vi "OP400ZP_SCANequipements.vi"(8 "Errin":errorcluster caption="errin", 10 "Chaîne":string="Log et conf\\Config.ini", 11 "pathin":path=path "D:/CODE/02 SLIM ZEN") -> (0 "errout":errorcluster={"status"=TRUE, "code"=0, "source"="PCAN_CHANNEL ILLEGAL"}, 1 "KO?":bool=TRUE, 4 "BT":refnum<visa-resource-name>, 6 "MX":refnum<visa-resource-name>)   [LabVIEW 2020]
doc: "Ce vi il détecte la presence des équipements"
uses:
  VG/VG_MX5060.vi
  VG/VG_BT3562.vi
  VG/VG_ARDUINO.vi
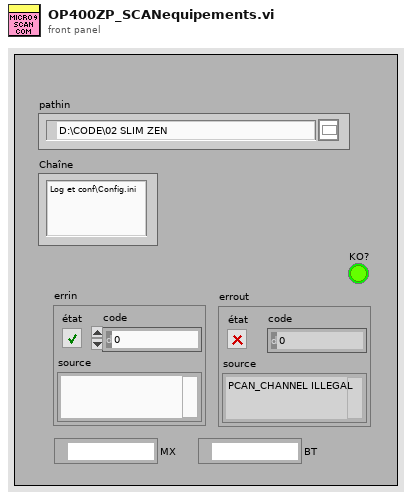
[diagram p1: front panel]
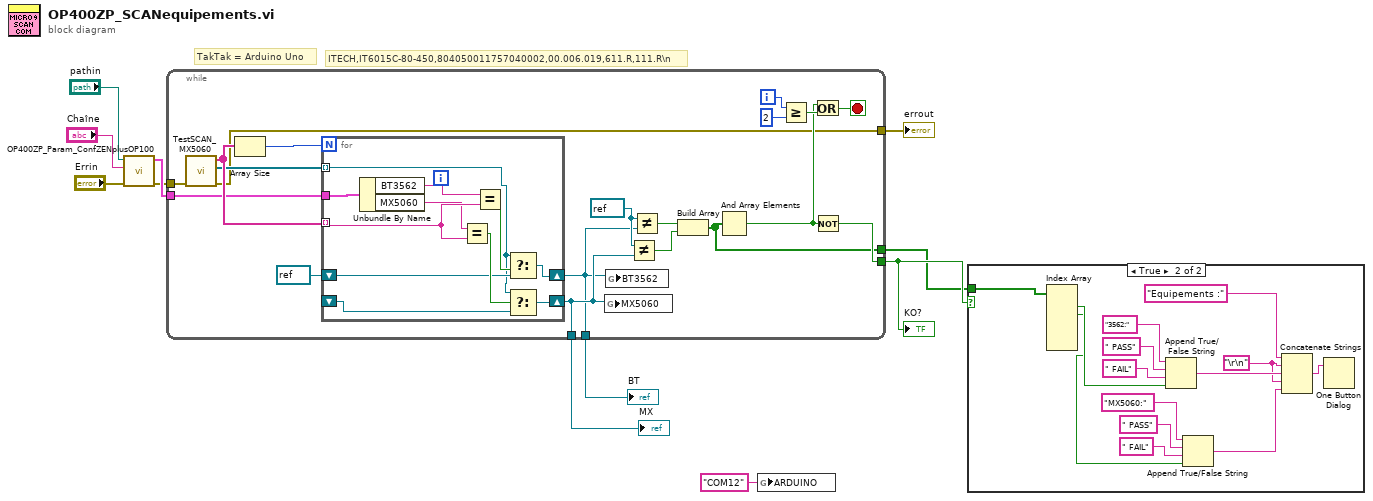
[diagram p0: block diagram]
diagram:
  # "TakTak = Arduino Uno"
  # "ITECH,IT6015C-80-450,804050011757040002,00.006.019,611.R,111.R\\n"
  n1 = call "OP400ZP_Param_ConfZENplusOP100.vi"("errin"="Errin", "Chaîne"="Chaîne", "pathin"="pathin") -> ("errout"=w8:errorcluster, "VISA OUT"=w9:cluster{"BT3562":string, "MX5060":string})  [unwired: 7 in]
  n2 = while {
    tunnel: w8 -> [w29]
    tunnel: [w24] -> w11
    tunnel: w9 -> [w21]
    tunnel: [w12] -> w10
    tunnel: [w18] -> w2
    tunnel: [w16] -> w4
    tunnel: [w15] -> w3
    i -> [w23]
    stop <- w26 stop-if-true
    w17 = refnum<visa-resource-name> refnum ("x")
    n3 = call "TestSCAN_MX5060.vi"("errin"=w29) -> ("error out"=w18:errorcluster, "Tableau 2"=w27:refnum<visa-resource-name>[], "Tableau"=w28:string[])  [unwired: 8 in]
    n4 = Array Size(array=w28) -> (size(s)=w30:i32)
    n5 = for {
      N: w30 -> [_]
      shift-right: [w40] -> w15
      shift-left: refnum<visa-resource-name> refnum ("VISA resource name out") -> [w34]
      tunnel: w28 -> [w37] mode=indexing
      tunnel: w27 -> [w31] mode=indexing
      tunnel: w21 -> [w39]
      shift-right: [w33] -> w16
      shift-left: _ -> [w32]
      n6 = Unbundle By Name(w39) -> ("BT3562"=w38:string, "MX5060"=w36:string)
      n7 = Equal?(x=w36, y=w37) -> (x = y?=w35:bool)
      n8 = Equal?(x=w38, y=w37) -> (x = y?=w41:bool)
      n9 = Select(t=w31, s=w41, f=w34) -> (s? t:f=w40:refnum<visa-resource-name>)
      n10 = Select(t=w31, s=w35, f=w32) -> (s? t:f=w33:refnum<visa-resource-name>)
    }
    n11 = global write "VG_MX5060.vi" "MX5060"(w16) -> ()
    n12 = global write "VG_BT3562.vi" "BT3562"(w15) -> ()
    n13 = Not Equal?(x=w17, y=w16) -> (x != y?=w13:bool)
    n14 = Not Equal?(x=w17, y=w15) -> (x != y?=w14:bool)
    n15 = Build Array(w14, w13) -> (w12:bool[])
    n16 = And Array Elements(Boolean array=w12) -> (logical AND=w19:bool)
    n17 = Greater Or Equal?(x=w23, y=2) -> (x >= y?=w25:bool)
    n18 = Or(x=w19, y=w25) -> (x .or. y?=w26:bool)
    n19 = Not(x=w19) -> (.not. x?=w24:bool)
  }
  "KO?" <- w11
  "errout" <- w2
  "MX" <- w4
  "BT" <- w3
  n20 = global write "VG_ARDUINO.vi" "ARDUINO"("COM12" ("ARDUINO")) -> ()
  n21 = case shown="True" w11 {
    tunnel: w10 -> [_ w51]
    frame False {
    }
    frame True {
      w48 = "\r\n"
      n22 = Index Array(array=w51) -> (element #1=w43:bool, element #2=w42:bool)  [unwired: 6 in, 4 out]
      n23 = Append True/False String(1:w43, 2:" FAIL" ("chaîne faux"), 3:" PASS" ("chaîne faux"), 4:"3562:" ("chaîne (\"\")")) -> (0:w53:string)
      n24 = Append True/False String(1:w42, 2:" FAIL" ("chaîne faux"), 3:" PASS" ("chaîne faux"), 4:"MX5060:" ("chaîne (\"\")")) -> (0:w44:string)
      n25 = Concatenate Strings("Equipements :" ("chaîne"), w48, w53, w48, w44) -> (w52:string)
      n26 = One Button Dialog(message=w52) -> ()  [unwired: 1 in, 1 out]
    }
  }
